vi "Write Max Qorf DVR.vi"(8 "error in (no error)":errorcluster, 10 "Max Qorf DVR":refnum<data-value>, 11 "Get Max Orifice Flow in":refnum<class "Get Max Orifice Flow.lvclass">) -> (0 "error out":errorcluster, 3 "Get Max Orifice Flow out":refnum<class "Get Max Orifice Flow.lvclass">)   [LabVIEW 2015, in "Get Max Orifice Flow.lvclass"]
uses:
  Get Max Orifice Flow.lvclass
  Get Max Orifice Flow.lvclass/Get Max Orifice Flow.ctl
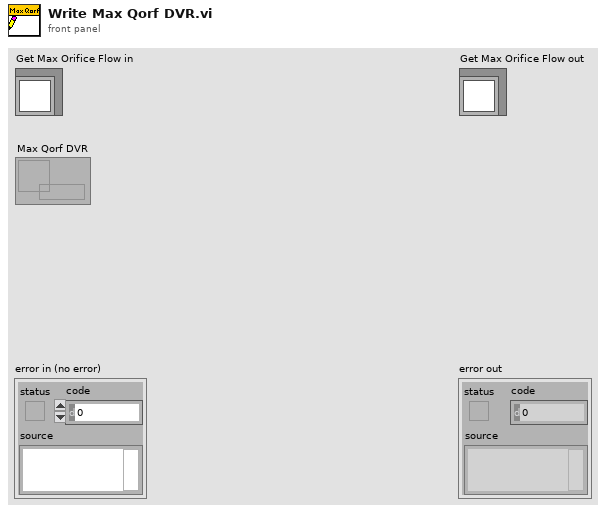
[diagram p1: front panel]
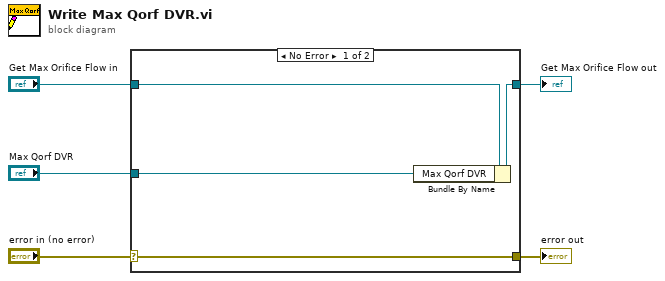
[diagram p0: block diagram]
diagram:
  n1 = case shown="No Error" "error in (no error)" {
    selector: "error in (no error)" -> [w9 w10]
    tunnel: [w9 w10] -> w4
    tunnel: [w7 w11] -> w2
    tunnel: "Get Max Orifice Flow in" -> [w8 w11]
    tunnel: "Max Qorf DVR" -> [w6 _]
    frame No Error {
      n2 = Bundle By Name(cluster=w8, "Max Qorf DVR"=w6) -> (w7:refnum<class "Get Max Orifice Flow.lvclass">)
    }
    frame Error {
    }
  }
  "error out" <- w4
  "Get Max Orifice Flow out" <- w2
